vi "PH_SSAC.PC Background Read.vi"(0 "i ref in":refnum<vi>, 2 "BG Read":bool, 5 "error IO":errorcluster) -> (14 "i ref in":refnum<vi>, 19 "error out":errorcluster)   [LabVIEW 2014, in "PH_SSAC.lvlib"]
uses:
  PH_SSAC.lvlib
  PH_SSAC.Background Data.ctl
  PH_SSAC.Signal Selector.ctl
  PH_Common/PH_Common.lvlib
panel:
  in  "Background Calibration Data":T1={"Date"="", "Time"="", "Frame Main"={"x"=0, "dx"=0, "y"=0, "dy"=0}, "dt [fs]"=0.0, "Calibration Factor [fs/pixel]"=0.0, "Signal"=array[1280 elements], "Frame Background"={"x"=0, "dx"=100, "y"=400, "dy"=250}}
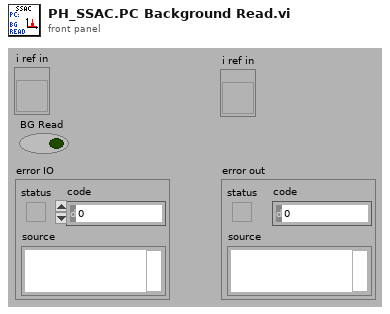
[diagram p1: front panel]
types:
  T1 = typedef "PH_SSAC.lvlib/PH_SSAC.Background Data.ctl" = cluster{"Date":string, "Time":string, "Frame Main":cluster{"x":u32, "dx":u32, "y":u32, "dy":u32}, "dt [fs]":dbl, "Calibration Factor [fs/pixel]":dbl, "Signal":dbl[], "Frame Background":cluster{"x":u32, "dx":u32, "y":u32, "dy":u32}}
  T2 = typedef "PH_SSAC.lvlib/PH_SSAC.i attribute.ctl" = cluster{"GUI Refs":cluster{"Delete":refnum<vi>, "Global On":refnum<vi>, "Cam Source":refnum<vi>, "Frame Main Signal":refnum<vi>, "Frame Background":refnum<vi>, "dt (Gauss smooth)":refnum<vi>, "Calibration Factor":refnum<vi>, "Background acquire":refnum<vi>, "Threshold":refnum<vi>, "Time evolution of mean pulse duration":refnum<vi>, "Mean Pulse Duration":refnum<vi>, "Main signal":refnum<vi>, "Current Pulse Duration":refnum<vi>, "Processed":refnum<vi>, "Saturation":refnum<vi>, "# for Average":refnum<vi>, "Position":refnum<vi>, "BG Status":refnum<vi>, "Save BG data":refnum<vi>, "Read BG Data":refnum<vi>, "Background Calibration Data":refnum<vi>}, "Images":cluster{"OP Image":T3, "GUI Image":T3, "PSDB Image":T3}, "Global On?":bool, "Frame Main":cluster{"x":u32, "dx":u32, "y":u32, "dy":u32}, "Frame Background":cluster{"x":u32, "dx":u32, "y":u32, "dy":u32}, "dt [fs]":dbl, "Calibration Factor [fs/pixel]":dbl, "Threshold":dbl, "Time evolution of mean pulse duration [fs]":dbl[], "Main Signal":cluster{"Time for Main":dbl[], "Signal":dbl[]}, "Processed":bool, "Current Pulse Duration [fs]":dbl, "# for Average":i32, "Position":i32, "Pulse Durations [fs]":dbl[], "BG":cluster{"Acquire?":bool, "Background Calibration Data":T1, "Save Data":bool}}
  T3 = typedef "IMAQ Image.ctl" = refnum<image>
  T4 = typedef "PH_SSAC.lvlib/PH_SSAC.Signal Selector.ctl" = enum16{"Main", "Background"}
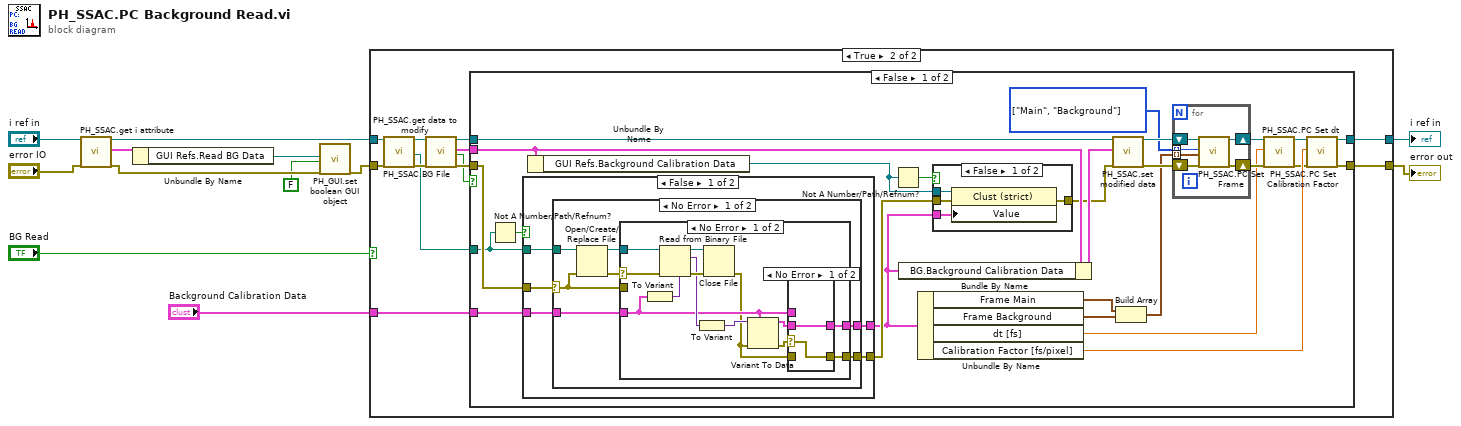
[diagram p0: block diagram]
diagram:
  n1 = call "PH_SSAC.get i attribute.vi"("i ref in"="i ref in", "error in (no error)"="error IO") -> ("i ref out"=w6:refnum<vi>, "i attribute"=w5:T2, "error out"=w7:errorcluster)  [unwired: 15 in]
  n2 = Unbundle By Name(w5) -> ("GUI Refs.Read BG Data"=w4:refnum<vi>)
  n3 = call "PH_GUI.set boolean GUI object.vi"("Boolean Knob GUI Ref"=w4, "Value"=FALSE, "error in (no error)"=w7) -> ("error out"=w2:errorcluster)  [unwired: 16 in]
  n4 = case shown="True" "BG Read" {
    tunnel: w6 -> [w13 w26]
    tunnel: [w13 w25] -> w11
    tunnel: [w14 w24] -> w10
    tunnel: w2 -> [w14 w23]
    tunnel: "Background Calibration Data" -> [_ w22]
    frame False {
    }
    frame True {
      n5 = call "PH_SSAC.BG File.vi"("i ref in"=w26, "error in"=w23) -> ("i ref out"=w21:refnum<vi>, "BG File"=w19:path, "error out"=w20:errorcluster)  [unwired: 15 in]
      n6 = call "PH_SSAC.get data to modify.vi"("i ref in"=w21, "error in (no error)"=w20) -> ("i ref out"=w18:refnum<vi>, "i attribute"=w15:T2, "timed out"=w16:bool, "error out"=w17:errorcluster)  [unwired: 14 in]
      n7 = case shown="False" w16 {
        tunnel: [w42 w100] -> w25
        tunnel: [w41 w99] -> w24
        tunnel: w22 -> [w52 _]
        tunnel: w18 -> [w50 w100]
        tunnel: w17 -> [w49 w99]
        tunnel: w19 -> [w27 _]
        tunnel: w15 -> [w47 _]
        frame False {
          w28 = T4[] [enum."Main", enum."Background"] items=["Main", "Background"]
          n8 = Not A Number/Path/Refnum?(number/path/refnum=w27) -> (NaN/Path/Refnum?=w51:bool)
          n9 = case shown="False" w51 {
            tunnel: [w68 w98] -> w44
            tunnel: w49 -> [w64 w98]
            tunnel: w52 -> [w67 w97]
            tunnel: [w66 w97] -> w40
            tunnel: w27 -> [w65 _]
            frame False {
              n10 = case shown="No Error" w64 {
                selector: w64 -> [w70 w96]
                tunnel: w65 -> [w74 _]
                tunnel: [w73 w96] -> w68
                tunnel: [w72 w95] -> w66
                tunnel: w67 -> [w69 w95]
                frame No Error {
                  n11 = Open/Create/Replace File(file path (use dialog)=w74, error in=w70) -> (refnum out=w75:refnum<file>, error out=w71:errorcluster)  [unwired: 4 in, 1 out]
                  n12 = case shown="No Error" w71 {
                    selector: w71 -> [w85 _]
                    tunnel: w75 -> [w88 _]
                    tunnel: [w77 w94] -> w73
                    tunnel: [w79 w93] -> w72
                    tunnel: w69 -> [w80 w93]
                    tunnel: w70 -> [_ w94]
                    frame No Error {
                      n13 = To Variant(anything=w80) -> (Variant=w82:variant)
                      n14 = Read from Binary File(5:w82, 8:w85, 11:w88) -> (0:w86:errorcluster, 2:w84:variant, 3:w87:refnum<file>)  [unwired: 3 in, 1 out]
                      n15 = To Variant(anything=w84) -> (Variant=w83:variant)
                      n16 = Close File(refnum=w87, error in=w86) -> (error out=w76:errorcluster)  [unwired: 1 out]
                      n17 = Variant To Data(error in=w76, type=w80, Variant=w83) -> (data=w78:T1, error out=w81:errorcluster)
                      n18 = case shown="No Error" w81 {
                        selector: w81 -> [w89 _]
                        tunnel: w80 -> [_ w92]
                        tunnel: [w90 w92] -> w79
                        tunnel: w78 -> [w90 _]
                        tunnel: [w89 w91] -> w77
                        tunnel: w76 -> [_ w91]
                        frame No Error {
                        }
                        frame Error {
                        }
                      }
                    }
                    frame Error {
                    }
                  }
                }
                frame Error {
                }
              }
            }
            frame True {
            }
          }
          n19 = Unbundle By Name(w47) -> ("GUI Refs.Background Calibration Data"=w45:refnum<vi>)
          n20 = Not A Number/Path/Refnum?(number/path/refnum=w45) -> (NaN/Path/Refnum?=w46:bool)
          n21 = Bundle By Name(cluster=w47, "BG.Background Calibration Data"=w40) -> (w48:T2)
          n22 = Unbundle By Name(w40) -> ("Frame Main"=w30:cluster{"x":u32, "dx":u32, "y":u32, "dy":u32}, "Frame Background"=w31:cluster{"x":u32, "dx":u32, "y":u32, "dy":u32}, "dt [fs]"=w32:dbl, "Calibration Factor [fs/pixel]"=w39:dbl)
          n23 = case shown="False" w46 {
            tunnel: w45 -> [w62 _]
            tunnel: w40 -> [w61 _]
            tunnel: w44 -> [w60 w63]
            tunnel: [w59 w63] -> w43
            frame False {
              n24 = property class="Clust (strict)"(reference=w62, error in=w60, "Value"=w61) -> (error out=w59:errorcluster)  [unwired: 1 out]
            }
            frame True {
            }
          }
          n25 = call "PH_SSAC.set modified data.vi"("i ref in"=w50, "i attribute"=w48, "error in (no error)"=w43) -> ("i ref out"=w37:refnum<vi>, "error out"=w38:errorcluster)  [unwired: 15 in]
          n26 = Build Array(w30, w31) -> (w29:cluster{"x":u32, "dx":u32, "y":u32, "dy":u32}[])
          n27 = for {
            tunnel: w28 -> [w56] mode=indexing
            tunnel: w29 -> [w53] mode=indexing
            shift-right: [w54] -> w34
            shift-left: w37 -> [w57]
            shift-right: [w55] -> w36
            shift-left: w38 -> [w58]
            n28 = call "PH_SSAC.PC Set Frame.vi"("i ref in"=w57, "Signal"=w56, "Frame"=w53, "error IO"=w58) -> ("i ref out"=w54:refnum<vi>, "error out"=w55:errorcluster)  [unwired: 14 in]
          }
          n29 = call "PH_SSAC.PC Set dt.vi"("i ref in"=w34, "dt"=w32, "error IO"=w36) -> ("i ref out"=w33:refnum<vi>, "error out"=w35:errorcluster)  [unwired: 15 in]
          n30 = call "PH_SSAC.PC Set Calibration Factor.vi"("i ref in"=w33, "Calibration Factor [fs/pixel]"=w39, "error IO"=w35) -> ("i ref out"=w42:refnum<vi>, "error out"=w41:errorcluster)  [unwired: 15 in]
        }
        frame True {
        }
      }
    }
  }
  "i ref in" <- w11
  "error out" <- w10
